vi "Disconnect.vi"(8 "error in (no error)":errorcluster, 11 "Database in":refnum<class "Database.lvclass">) -> (0 "error out":errorcluster, 3 "Database out":refnum<class "Database.lvclass">)   [LabVIEW 2014, in "Database.lvclass"]
uses:
  Database.lvclass
  Database.lvclass/Database.ctl
  <vilib>/addons/database/NI_Database_API.lvlib
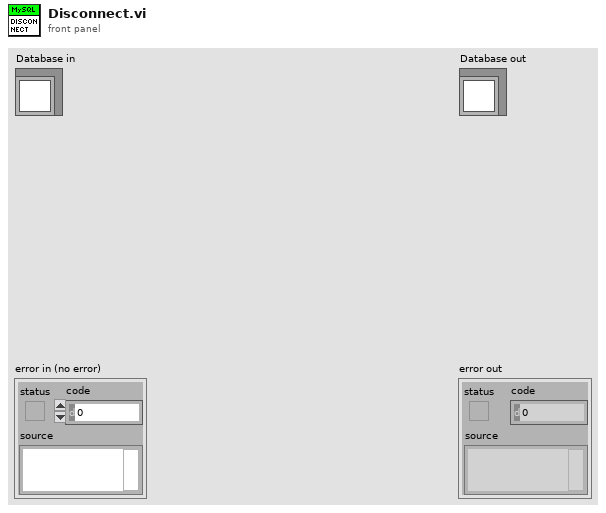
[diagram p1: front panel]
types:
  T1 = typedef "NI_Database_API.lvlib/Conn ObjectReference.ctl" = refnum<k1>
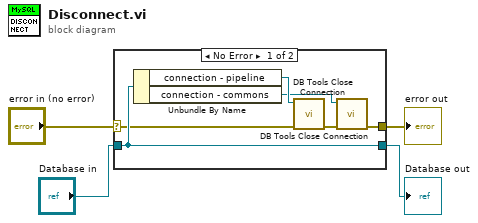
[diagram p0: block diagram]
diagram:
  n1 = case shown="No Error" "error in (no error)" {
    selector: "error in (no error)" -> [w8 w12]
    tunnel: [w6 w12] -> w3
    tunnel: [w10 w11] -> w1
    tunnel: "Database in" -> [w10 w11]
    frame No Error {
      n2 = Unbundle By Name(w10) -> ("connection - pipeline"=w9:T1, "connection - commons"=w5:T1)
      n3 = call <vilib>:"DB Tools Close Connection.vi"("error in (no error)"=w8, "connection reference"=w9) -> ("error out"=w7:errorcluster)  [unwired: 5 in]
      n4 = call <vilib>:"DB Tools Close Connection.vi"("error in (no error)"=w7, "connection reference"=w5) -> ("error out"=w6:errorcluster)  [unwired: 5 in]
    }
    frame Error {
    }
  }
  "error out" <- w3
  "Database out" <- w1
